vi "Radiation.vi"() -> ()   [LabVIEW 2012]
uses:
  <vilib>/Math Plots/2D Math Plots/2D Compass/2D Compass XCtrl/2D Compass.xctl
  <vilib>/Math Plots/2D Math Plots/2D Compass/2D Compass Datatype/Public/Plot Helper (Vector).vi
  <vilib>/Utility/file.llb/Write To Spreadsheet File (DBL).vi
  <vilib>/Math Plots/2D Math Plots/2D Compass/2D Compass Datatype/2D Compass Datatype.lvclass
panel:
  in  "?":bool
  out "?":dbl[][](array[numeric])
  in  "?":bool
  out "2D Compass":refnum<class "2D Plot Datatype.lvclass">[](xcontrol)
  in  "E [MeV]":dbl(slide) min=0.0 max=2.0 scale=0.0..2.0
  in  "0-360":dbl(knob) min=0.0 max=360.0 step=1.0 scale=0.0..360.0
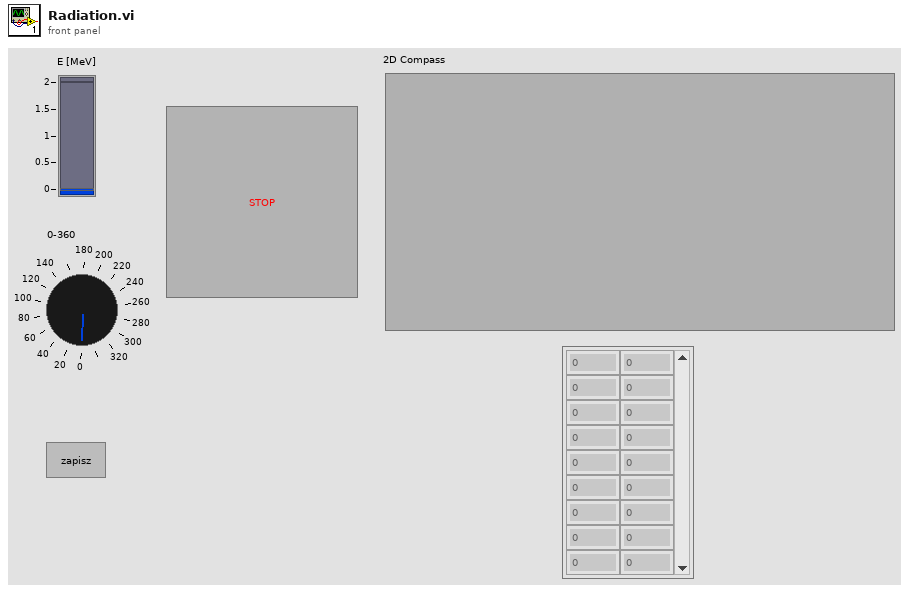
[diagram p1: front panel]
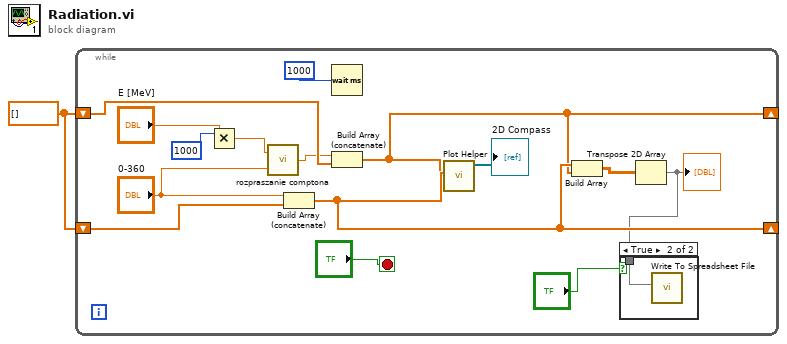
[diagram p0: block diagram]
diagram:
  w1 = dbl[] []
  n1 = while {
    shift-right: [w5] -> _
    shift-left: w1 -> [w9]
    shift-right: [w6] -> _
    shift-left: w1 -> [w8]
    stop <- "?" stop-if-true
    n2 = Multiply(x=1000, y="E [MeV]") -> (x*y=w14:dbl)
    n3 = call "rozpraszanie comptona.vi"("theta"="0-360", "E"=w14) -> ("E_compt"=w7:dbl)
    n4 = Build Array (concatenate)("0-360", w8) -> (w6:dbl[])
    n5 = Wait (ms)(milliseconds to wait=1000) -> ()  [unwired: 1 out]
    n6 = Build Array (concatenate)(w7, w9) -> (w5:dbl[])
    n7 = call-poly <vilib>:"Plot Helper.vi"("radius vector"=w5, "theta vector"=w6) -> ("2D Plot Class Obj Array out"=→"2D Compass":refnum<class "2D Plot Datatype.lvclass">[])  [unwired: 2 in, 7 out]
    n8 = Build Array(w6, w5) -> (w4:dbl[][])
    n9 = Transpose 2D Array(2D array=w4) -> (transposed array=w2:dbl[][])
    "?" <- w2
    n10 = case shown="True" "?" {
      tunnel: w2 -> [_ w17]
      frame False {
      }
      frame True {
        n11 = call-poly <vilib>:"Write To Spreadsheet File.vi"("2D data"=w17) -> ()  [unwired: 7 in, 1 out]
      }
    }
  }
